vi "Quaternion_Times.vi"(9 "Other Quaternion":T1={"R"=1.0, "V"=[0.0, 0.0, 0.0]}, 11 "Quaternion":T1={"R"=1.0, "V"=[0.0, 0.0, 0.0]}) -> (3 "Times":T1={"R"=1.0, "V"=[0.0, 0.0, 0.0]})   [LabVIEW 2019, in "Trajectory_Library.lvlib"]
doc: "Convenience constructors that takes in x and y values directly instead of having to construct a Translation2d.\n\nParameters:\n - X- The x component of the translational component of the pose.\n - Y - The y component of the translational component of the pose.\n - Rotation (Heading) - The rotational component of the pose.\n\nReturns:\n - OUT POSE - Output POSE"
uses:
  Trajectory_Library.lvlib
  QUATERNION.ctl
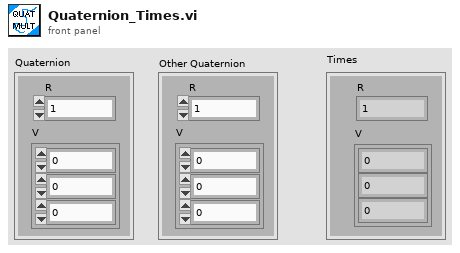
[diagram p1: front panel]
types:
  T1 = typedef "Trajectory_Library.lvlib/QUATERNION.ctl" = cluster{"R":dbl, "V":dbl[]}
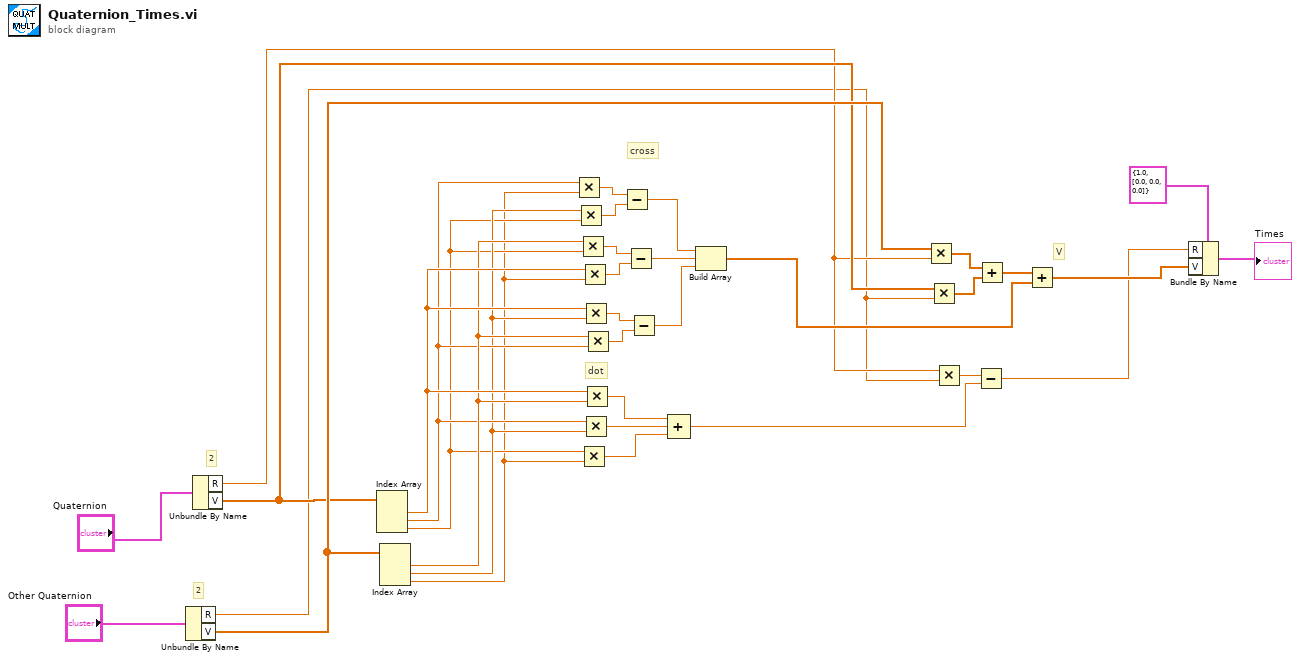
[diagram p0: block diagram]
diagram:
  # "V"
  # "2"
  # "2"
  # "dot"
  # "cross"
  n1 = Unbundle By Name("Other Quaternion") -> ("R"=w5:dbl, "V"=w17:dbl[])
  n2 = Unbundle By Name("Quaternion") -> ("R"=w6:dbl, "V"=w16:dbl[])
  n3 = Index Array(array=w16) -> (element #1=w26:dbl, element #2=w24:dbl, element #3=w22:dbl)  [unwired: 3 in]
  n4 = Index Array(array=w17) -> (element #1=w25:dbl, element #2=w23:dbl, element #3=w21:dbl)  [unwired: 3 in]
  n5 = Multiply(x=w24, y=w21) -> (x*y=w30:dbl)
  n6 = Multiply(x=w23, y=w22) -> (x*y=w31:dbl)
  n7 = Multiply(x=w25, y=w22) -> (x*y=w32:dbl)
  n8 = Multiply(x=w22, y=w21) -> (x*y=w18:dbl)
  n9 = Multiply(x=w26, y=w21) -> (x*y=w33:dbl)
  n10 = Multiply(x=w26, y=w23) -> (x*y=w27:dbl)
  n11 = Multiply(x=w24, y=w23) -> (x*y=w19:dbl)
  n12 = Multiply(x=w26, y=w25) -> (x*y=w20:dbl)
  n13 = Multiply(x=w25, y=w24) -> (x*y=w28:dbl)
  n14 = Subtract(x=w30, y=w31) -> (x-y=w12:dbl)
  n15 = Subtract(x=w32, y=w33) -> (x-y=w11:dbl)
  n16 = Subtract(x=w27, y=w28) -> (x-y=w10:dbl)
  n17 = Compound Arithmetic op=ADD(w20, w19, w18) -> (w3:dbl)
  n18 = Build Array(w12, w11, w10) -> (w9:dbl[])
  n19 = Multiply(x=w17, y=w6) -> (x*y=w15:dbl[])
  n20 = Multiply(x=w16, y=w5) -> (x*y=w14:dbl[])
  n21 = Multiply(x=w6, y=w5) -> (x*y=w4:dbl)
  n22 = Subtract(x=w4, y=w3) -> (x-y=w2:dbl)
  n23 = Add(x=w15, y=w14) -> (x+y=w13:dbl[])
  n24 = Add(x=w13, y=w9) -> (x+y=w7:dbl[])
  n25 = Bundle By Name(cluster=T1 {"R"=1.0, "V"=[0.0, 0.0, 0.0]} ("sumPOSE"), "R"=w2, "V"=w7) -> (→"Times":T1)
